vi "notImaging.vi"(8 "error in (no error)":errorcluster, 9 "command_stopImageCapture":T1, 10 "model in":refnum<class "IModel.lvclass">, 11 "NotImagingState in":refnum<class "NotImagingState.lvclass">) -> (0 "error out":errorcluster, 2 "model out":refnum<class "IModel.lvclass">, 3 "NotImagingState out":refnum<class "NotImagingState.lvclass">)   [LabVIEW 2016, in "States.lvlib" / "NotImagingState.lvclass"]
uses:
  NotImagingState.lvclass
  IModel/IModel.lvclass
  ts_sallv_sedspectrometer/DataTypes/command_stopImageCapture.ctl
  EnabledState.lvclass
  ts_sallv_sedspectrometer/SALLV_sedSpectrometer.lvlib
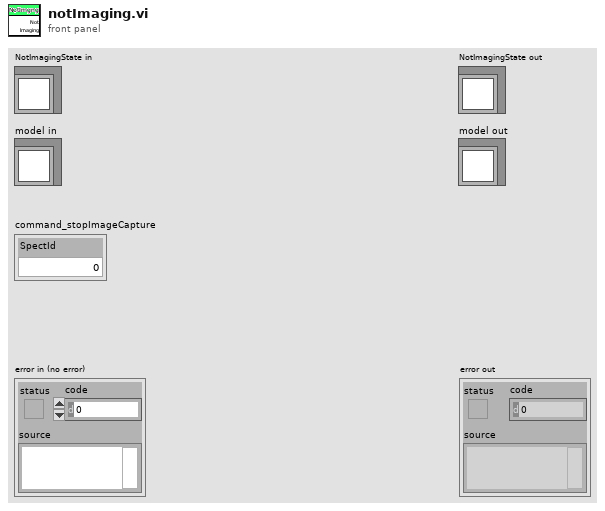
[diagram p1: front panel]
types:
  T1 = typedef "SALLV_sedSpectrometer.lvlib/command_stopImageCapture.ctl" = cluster{"SpectId":u16}
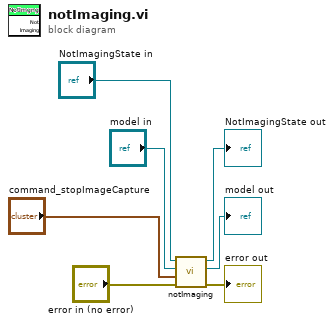
[diagram p0: block diagram]
diagram:
  n1 = call-parent "notImaging.vi"("error in (no error)"="error in (no error)", "command_stopImageCapture"="command_stopImageCapture", "model in"="model in", "State in"="NotImagingState in") -> ("error out"=→"error out":errorcluster, "model out"=→"model out":refnum<class "IModel.lvclass">, "State out"=→"NotImagingState out":refnum<class "NotImagingState.lvclass">)  [unwired: 5 in]
